vi "Get MenuItemList.vi"(8 "error in (no error)":errorcluster, 11 "MenuCol in":refnum<class "MenuCol.lvclass">) -> (0 "error out":errorcluster, 2 "MenuItemList":string[](array[string])=["<No Items Defined>"], 3 "MenuCol out":refnum<class "MenuCol.lvclass">)   [LabVIEW 2013, in "MenuCol.lvclass"]
uses:
  MenuCol.lvclass
  MenuCol.lvclass/MenuCol.ctl
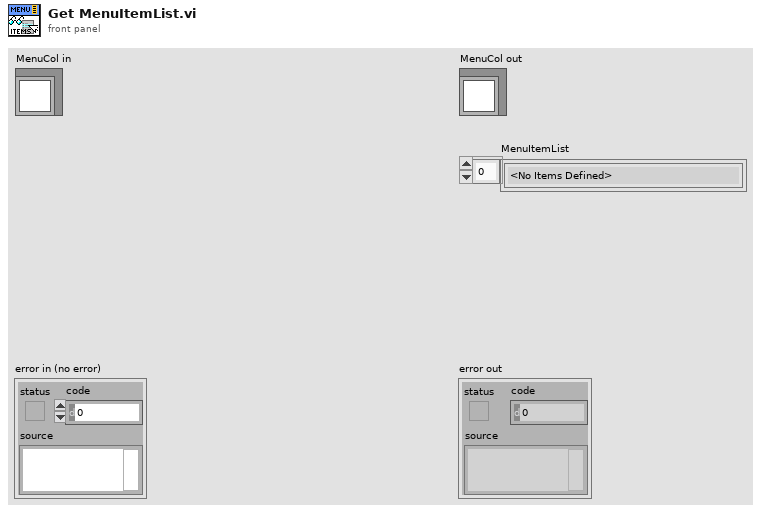
[diagram p1: front panel]
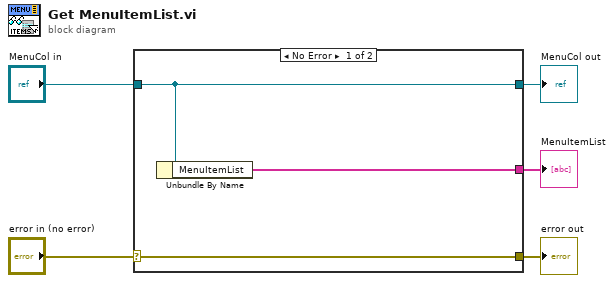
[diagram p0: block diagram]
diagram:
  n1 = case shown="No Error" "error in (no error)" {
    selector: "error in (no error)" -> [w8 w9]
    tunnel: [w8 w9] -> w4
    tunnel: [w7 w10] -> w2
    tunnel: "MenuCol in" -> [w7 w10]
    tunnel: [w6 _] -> w1
    frame No Error {
      n2 = Unbundle By Name(w7) -> ("MenuItemList"=w6:string[])
    }
    frame Error {
    }
  }
  "error out" <- w4
  "MenuCol out" <- w2
  "MenuItemList" <- w1
